vi "compute_CA.vi"(1 "additional vol. [ml]":dbl, 3 "pipette vol. [ml]":dbl, 4 "calibration vol. [ml]":dbl, 5 "mols in Cal-volume":dbl, 6 "ItemNames":string[][](array[string])) -> (0 "Array":string[][](array[string]))   [LabVIEW 2013]
doc: "Das VI berechnet die CAL-Amlounts in der CAL-bottle und die CAL-Amounts in der Pipette"
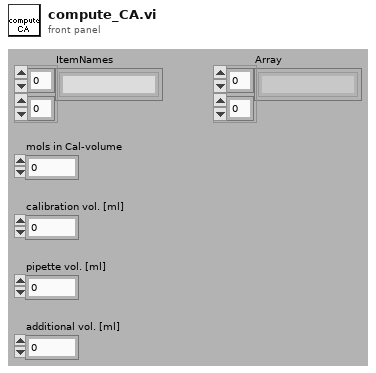
[diagram p1: front panel]
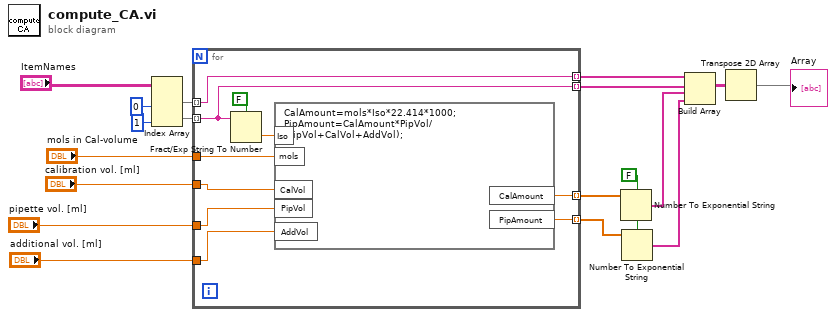
[diagram p0: block diagram]
diagram:
  w12 = FALSE ("use system decimal point (T)")
  n1 = Index Array(array="ItemNames", index (col) #1=0 ("disabled index (col)"), index (col) #2=1 ("index (col)")) -> (element #1=w8:string[], element #2=w7:string[])  [unwired: 2 in]
  n2 = for {
    tunnel: "mols in Cal-volume" -> [w26]
    tunnel: "pipette vol. [ml]" -> [w24]
    tunnel: "calibration vol. [ml]" -> [w25]
    tunnel: "additional vol. [ml]" -> [w23]
    tunnel: [w22] -> w10 mode=indexing
    tunnel: [w21] -> w11 mode=indexing
    tunnel: w7 -> [w19] mode=indexing
    tunnel: w8 -> [w20] mode=indexing
    tunnel: [w20] -> w9 mode=indexing
    tunnel: [w19] -> w17 mode=indexing
    n3 = Fract/Exp String To Number(use system decimal point (T)=FALSE, string=w19) -> (number=w27:dbl)  [unwired: 2 in, 1 out]
    n4 = formula code="CalAmount=mols*Iso*22.414*1000;\nPipAmount=CalAmount*PipVol/(PipVol+CalVol+AddVol);"("Iso"=w27, "mols"=w26, "PipVol"=w24, "CalVol"=w25, "AddVol"=w23) -> ("PipAmount"=w21:dbl, "CalAmount"=w22:dbl)
  }
  n5 = Number To Exponential String(number=w10, 1:w12) -> (E-format string=w13:string[])  [unwired: 2 in]
  n6 = Number To Exponential String(number=w11, 1:w12) -> (E-format string=w14:string[])  [unwired: 2 in]
  n7 = Build Array(w9, w17, w13, w14) -> (w15:string[][])
  n8 = Transpose 2D Array(2D array=w15) -> (transposed array=→"Array":string[][])
